vi "Knife_Edge_Scan_Parameters.vi"(0 "VISA Ressource in":refnum<visa-resource-name>="COM17", 1 "Axis":u16(ring) items=["Detector", "X-Rays", "Vertical", "In-Plain", "Vertical (with tilt)"], 5 "Scan Range (mum)":dbl=100.0, 7 "Nr. of Steps":u32=10, 9 "Z tilt (angle)":dbl, 11 "error in (no error)":errorcluster, 12 "Echo Mode":i32) -> (2 "V_max 1/3 and 2":i32[](array[numeric]), 3 "angle":dbl, 4 "VISA ressource out":refnum<visa-resource-name>, 6 "micron steps":dbl[](array[numeric]), 8 "single steps 1":i32[](array[numeric]), 10 "single steps 2":i32[](array[numeric]), 13 "Array Lengths equal?":bool, 14 "move time (ms)":u32, 15 "error out":errorcluster={"status"=FALSE, "code"=1073676294, "source"="VISA Read in write_read.vi"})   [LabVIEW 2018]
uses:
  ConversionAndInformation/Unit_Control.ctl
  MCode_LV_86/Set Parameter.ctl
panel:
  out "delta angle":dbl
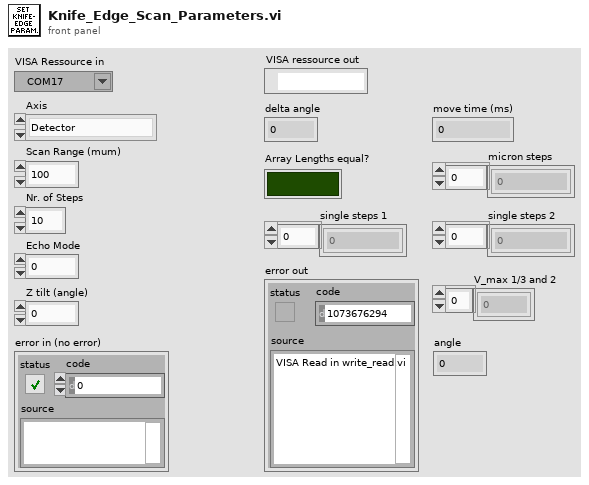
[diagram p1: front panel]
types:
  T1 = typedef "Unit_Control.ctl" = enum16{"Angle (Degrees)", "Rad", "Angle [TMC]", "Microsteps [TMC]", "Inches", "Nanometer", "Meter", "Centimeter", "Millimeter", "Micron"}
  T2 = typedef "Set Parameter.ctl" = enum16{"Acceleration (A)", "Baud Rate (BD)", "Counter 1 (C1)", "Counter 2 (C2)", "Control C Software Reset (CE)", "Check Sum Enable (CK)", "Clock Mode (CM)", "Clock Mode Ratio (CR)", "Clock Mode Out Step Width (CW)", "Deceleration (D)", "Digital Filtering, Input 1 (D1)", "Digital Filtering, Input 2 (D2)", "Digital Filtering, Input 3 (D3)", "Digital Filtering, Input 4 (D4)", "Digital Filtering, Input 5 (D5)", "Digital Filtering, Input 9 (D9)", "Digital Filtering, Input 10 (D10)", "Digital Filtering, Input 11 (D11)", "Digital Filtering, Input 12 (D12)", "Deadband (DB)", "Decrement Variable (DC)", "Enable/Disable Drive (DE)", "Device Name (DN)", "End Program Execution (E)", "Encoder Function Enable (EE)", "Error Flag (EF)", "Encoder Lines (EL)", "Echo Mode (EM)", "Error Value (ER)", "Escape (ES)", "Execute Program at Address (EX)", "Firmware Version (VR)", "Hold (H)", "Hold Current (HC)", "Hold Current Delay Time (HI)", "Home to Encoder Index (HM)", "Home to Home Switch (HT)", "Increment Variable (IC)", "Initialize Parameters to NVM (IP)", "Input into Variable (IV)", "Jog Enable (JE)", "Limit Stop Mode (LM)", "Move Absolute (MA)", "Move Relative (MR)", "MicroStepping Select (MS)", "Motor Settling Delay Time (MT)", "Moving [Flag] (MV)", "Output 1 (O1)", "Output 2 (O2)", "Output 3 (O3)", "Output 4 (O4)", "Output 9 (O9)", "Output 10 (O10)", "Output 11 (O11)", "Output 12 (O12)", "Output High Byte (9-12) (OH)", "Output Low Byte (1-4) (OL)", "Output Total (1-4 and 9-12) (OT)", "Position (P)", "Position Maintenance (PM)", "Party Mode (PY)", "Register 1 (R1)", "Register 2 (R2)", "Register 3 (R3)", "Register 4 (R4)", "Reset Error(\\03)", "Run Current (RC)", "Stall Factor (SF)", "Slew (SL)", "Stall Mode Set (SM)", "Upgrade Firmware (UG)", "Velocity Initial (VI)", "Velocity Maximum (VM)", "Current1 (I1)", "Current2 (I2)", "Current3 (I3)", "Current4 (I4)", "Current5 (I5)", "Current6 (I6)", "Save (S)"}
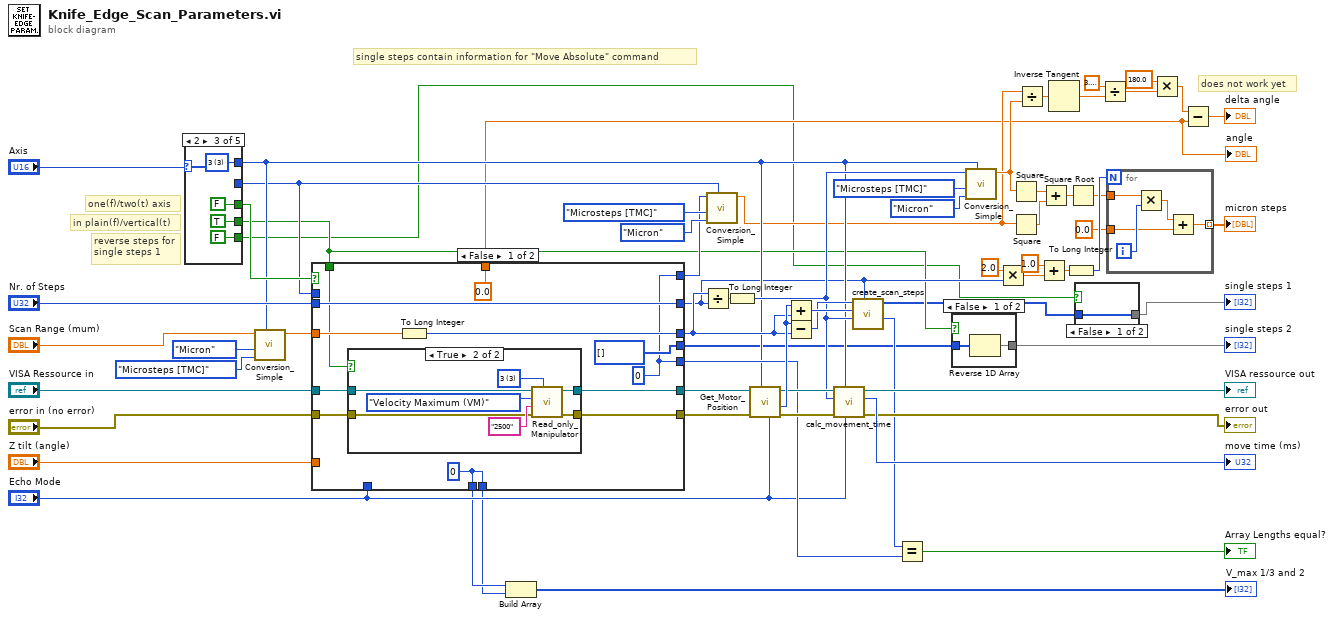
[diagram p0: block diagram]
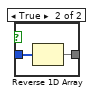
[diagram p2: hidden frame]
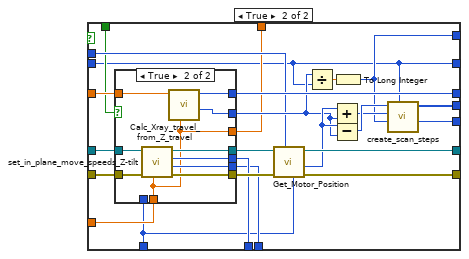
[diagram p5: hidden frame]
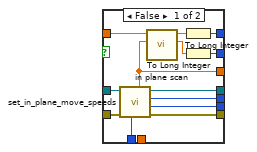
[diagram p6: hidden frame]
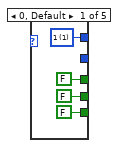
[diagram p7: hidden frame]
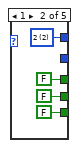
[diagram p8: hidden frame]
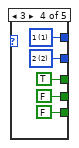
[diagram p9: hidden frame]
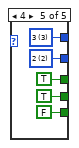
[diagram p10: hidden frame]
diagram:
  # "single steps contain information for \"Move Absolute\" command"
  # "reverse steps for\nsingle steps 1"
  # "does not work yet"
  # "in plain(f)/vertical(t)"
  # "one(f)/two(t) axis"
  n1 = case shown="2" "Axis" {
    tunnel: [w69 w73 w77 w82 w87] -> w36
    tunnel: [_ _ _ w81 w86] -> w33
    tunnel: [FALSE FALSE FALSE TRUE TRUE] -> w44
    tunnel: [FALSE FALSE TRUE FALSE TRUE] -> w5
    tunnel: [FALSE FALSE FALSE FALSE FALSE] -> w1
    frame 0, Default {
      w69 = u16 1 items=["none", "1", "2", "3", "4", "all"] ("Motor")
    }
    frame 1 {
      w73 = u16 2 items=["none", "1", "2", "3", "4", "all"] ("Motor")
    }
    frame 2 {
      w77 = u16 3 items=["none", "1", "2", "3", "4", "all"] ("Motor")
    }
    frame 3 {
      w81 = u16 2 items=["none", "1", "2", "3", "4", "all"] ("Motor")
      w82 = u16 1 items=["none", "1", "2", "3", "4", "all"] ("Motor")
    }
    frame 4 {
      w86 = u16 2 items=["none", "1", "2", "3", "4", "all"] ("Motor")
      w87 = u16 3 items=["none", "1", "2", "3", "4", "all"] ("Motor")
    }
  }
  n2 = call "Conversion_Simple.vi"("Motor"=w36, "Output Unit"=Unit_Control."Microsteps [TMC]", "Input Unit"=Unit_Control."Micron", "Input"="Scan Range (mum)") -> ("Output"=w57:dbl)  [unwired: 6 in, 1 out]
  n3 = case shown="False" w44 {
    tunnel: w57 -> [w98 w132]
    tunnel: [w91 w131] -> w56
    tunnel: [w89 w130] -> w55
    tunnel: [w99 w127] -> w16
    tunnel: [w99 w126] -> w15
    tunnel: [i32[] [] ("single steps") w122] -> w7
    tunnel: [w97 w120] -> w53
    tunnel: [w94 w118] -> w52
    tunnel: w33 -> [_ w117]
    tunnel: "Nr. of Steps" -> [w95 w109]
    tunnel: "VISA Ressource in" -> [w92 w116]
    tunnel: "error in (no error)" -> [w90 w115]
    tunnel: "Echo Mode" -> [_ w112]
    tunnel: w5 -> [w88 w114]
    tunnel: "Z tilt (angle)" -> [_ w113]
    tunnel: [w95 w109] -> w8
    tunnel: [w94 w111] -> w32
    tunnel: [0.0 w110] -> w4
    frame False {
      w94 = 0 ("array length")
      w99 = 0 ("V_max Motor 3")
      n4 = case shown="True" w88 {
        tunnel: w92 -> [w101 w106]
        tunnel: [w101 w105] -> w91
        tunnel: w90 -> [w100 w104]
        tunnel: [w100 w103] -> w89
        frame False {
        }
        frame True {
          w107 = u16 3 items=["none", "1", "2", "3", "4", "all"] ("Motor")
          n5 = call "Read_only_Manipulator.vi"("Motor"=w107, "error in (no error)"=w104, "Value"="2500", "Command"=Set_Parameter."Velocity Maximum (VM)", "VISA resource name"=w106) -> ("error out"=w103:errorcluster, "VISA ressource out"=w105:refnum<visa-resource-name>)  [unwired: 3 in, 2 out]
        }
      }
      n6 = To Long Integer(number=w98) -> (32bit integer=w97:i32)
    }
    frame True {
      n7 = case shown="True" w114 {
        tunnel: w132 -> [w145 w149]
        tunnel: [w144 w153] -> w129
        tunnel: [w143 w152] -> w128
        tunnel: [w142 w151] -> w127
        tunnel: [w141 w150] -> w126
        tunnel: [w138 w148] -> w120
        tunnel: [w137 w147] -> w119
        tunnel: w116 -> [w136 w155]
        tunnel: w115 -> [w135 w154]
        tunnel: w112 -> [w134 _]
        tunnel: w113 -> [_ w146]
        tunnel: [w133 w146] -> w110
        frame False {
          n8 = call "set_in_plane_move_speeds.vi"("Echo Mode"=w134, "error in (no error)"=w135, "VISA resource name"=w136) -> ("error out"=w143:errorcluster, "V_max Motor 2"=w141:i32, "V_max Motor 1"=w142:i32, "VISA ressource out"=w144:refnum<visa-resource-name>, "Angle Sample Holder"=w133:dbl)  [unwired: 4 in]
          n9 = call "in plane scan.vi"("angle (degrees)"=w133, "v total"=w145) -> ("v_y"=w140:dbl, "v_x"=w139:dbl)  [unwired: 4 in, 4 out]
          n10 = To Long Integer(number=w139) -> (32bit integer=w138:i32)
          n11 = To Long Integer(number=w140) -> (32bit integer=w137:i32)
        }
        frame True {
          n12 = call "set_in_plane_move_speeds_Z-tilt.vi"("Z tilt (angle)"=w146, "error in (no error)"=w154, "VISA resource name"=w155) -> ("error out"=w152:errorcluster, "V_max Motor 2"=w150:i32, "V_max Motor 3"=w151:i32, "VISA ressource out"=w153:refnum<visa-resource-name>)  [unwired: 5 in]
          n13 = call "Calc_Xray_travel_from_Z_travel.vi"("Z tilt (degrees)"=w146, "Z travel (steps)"=w149) -> ("X-ray travel (steps)"=w147:i32, "Z travel (steps)"=w148:i32)  [unwired: 8 in]
        }
      }
      n14 = call "Get_Motor_Position.vi"("Echo Mode (2)"=w112, "Motor In"=w117, "error in (no error)"=w128, "VISA resource name"=w129) -> ("error out"=w130:errorcluster, "Position (Steps)"=w123:i32, "VISA ressource out"=w131:refnum<visa-resource-name>)  [unwired: 4 in, 1 out]
      n15 = Divide(x=w119, y=w109) -> (x/y=w121:dbl)
      n16 = Add(x=w123, y=w119) -> (x+y=w124:i32)
      n17 = Subtract(x=w123, y=w119) -> (x-y=w125:i32)
      n18 = To Long Integer(number=w121) -> (32bit integer=w111:i32)
      n19 = call "create_scan_steps.vi"("number of steps"=w109, "step"=w111, "stop"=w124, "start"=w125) -> ("array length"=w118:i32, "single steps"=w122:i32[])  [unwired: 6 in]
    }
  }
  "angle" <- w4
  n20 = Build Array(w16, w15) -> (→"V_max 1/3 and 2":i32[])
  n21 = Divide(x=w53, y=w8) -> (x/y=w54:dbl)
  n22 = call "Conversion_Simple.vi"("Motor"=w33, "Output Unit"=Unit_Control."Micron", "Input Unit"=Unit_Control."Microsteps [TMC]", "Input"=w32) -> ("Output"=w17:dbl)  [unwired: 6 in, 1 out]
  n23 = To Long Integer(number=w54) -> (32bit integer=w37:i32)
  n24 = call "Get_Motor_Position.vi"("Echo Mode (2)"="Echo Mode", "Motor In"=w36, "error in (no error)"=w55, "VISA resource name"=w56) -> ("error out"=w60:errorcluster, "Position (Steps)"=w61:i32, "VISA ressource out"=w59:refnum<visa-resource-name>)  [unwired: 4 in, 1 out]
  n25 = Add(x=w61, y=w53) -> (x+y=w65:i32)
  n26 = Subtract(x=w61, y=w53) -> (x-y=w64:i32)
  n27 = call "calc_movement_time.vi"("Echo Mode"="Echo Mode", "Motor"=w36, "error in (no error)"=w60, "steps"=w37, "VISA ressource in"=w59) -> ("error out"=→"error out":errorcluster, "move time (ms)"=→"move time (ms)":u32, "VISA ressource out"=→"VISA ressource out":refnum<visa-resource-name>)  [unwired: 3 in, 1 out]
  n28 = call "create_scan_steps.vi"("number of steps"=w8, "step"=w37, "stop"=w65, "start"=w64) -> ("array length"=w40:i32, "single steps"=w3:i32[])  [unwired: 6 in]
  n29 = Equal?(x=w40, y=w52) -> (x = y?=→"Array Lengths equal?":bool)
  n30 = case shown="False" w5 {
    tunnel: w7 -> [w157 w158]
    tunnel: [w156 w158] -> w6
    frame False {
      n31 = Reverse 1D Array(array=w157) -> (reversed array=w156:i32[])
    }
    frame True {
    }
  }
  "single steps 2" <- w6
  n32 = call "Conversion_Simple.vi"("Motor"=w36, "Output Unit"=Unit_Control."Micron", "Input Unit"=Unit_Control."Microsteps [TMC]", "Input"=w37) -> ("Output"=w18:dbl)  [unwired: 6 in, 1 out]
  n33 = Multiply(x=2.0, y=w8) -> (x*y=w26:dbl)
  n34 = Square(x=w18) -> (x^2=w31:dbl)
  n35 = Square(x=w17) -> (x^2=w30:dbl)
  n36 = Divide(x=w17, y=w18) -> (x/y=w19:dbl)
  n37 = Add(x=1.0, y=w26) -> (x+y=w24:dbl)
  n38 = Add(x=w31, y=w30) -> (x+y=w29:dbl)
  n39 = Inverse Tangent(1:w19) -> (0:w12:dbl)
  n40 = To Long Integer(number=w24) -> (32bit integer=w23:i32)
  n41 = Square Root(x=w29) -> (sqrt(x)=w21:dbl)
  n42 = case shown="False" w1 {
    tunnel: w3 -> [w159 w161]
    tunnel: [w159 w160] -> w2
    frame False {
    }
    frame True {
      n43 = Reverse 1D Array(array=w161) -> (reversed array=w160:i32[])
    }
  }
  "single steps 1" <- w2
  n44 = Divide(x=3.141592653589793, y=w12) -> (x/y=w11:dbl)
  n45 = for {
    N: w23 -> [_]
    tunnel: 0.0 -> [w164]
    tunnel: w21 -> [w166]
    tunnel: [w162] -> w20 mode=indexing
    i -> [w165]
    n46 = Multiply(x=w166, y=w165) -> (x*y=w163:dbl)
    n47 = Add(x=w163, y=w164) -> (x+y=w162:dbl)
  }
  "micron steps" <- w20
  n48 = Multiply(x=180.0 ("y"), y=w11) -> (x*y=w9:dbl)
  n49 = Subtract(x=w9, y=w4) -> (x-y=→"delta angle":dbl)
